vi "Read DC Output.vi"(8 "error in (no error)":errorcluster, 11 "VISA resource name":refnum<visa-resource-name>) -> (0 "error out":errorcluster, 1 "Actual DC Current Level (A)":dbl format="%.4g", 2 "Actual DC Voltage Level (V)":dbl format="%.4g", 3 "VISA resource name out":refnum<visa-resource-name>)   [LabVIEW 2015, in "BK Precision 983X Series.lvlib"]
doc: "Returns the actual DC voltage level and actual DC current level."
uses:
  <instrlib>/BK Precision 983X Series/BK Precision 983X Series.lvlib
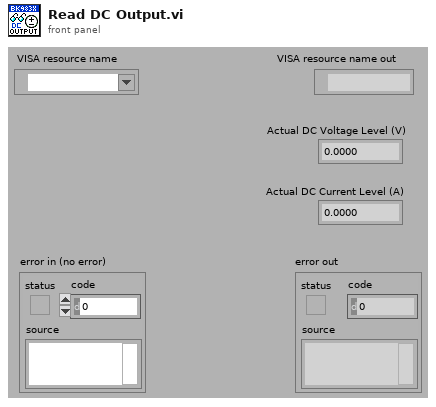
[diagram p1: front panel]
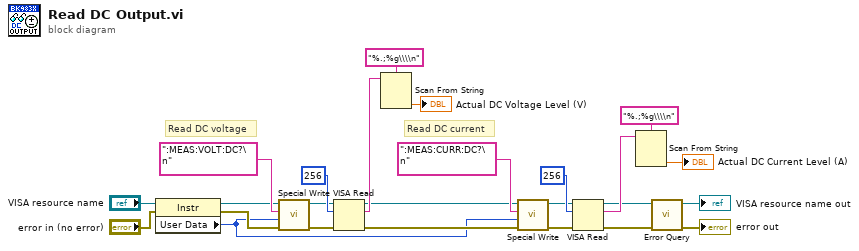
[diagram p0: block diagram]
diagram:
  # "Read DC current"
  # "Read DC voltage"
  n1 = property class="Instr"(reference="VISA resource name", error in="error in (no error)") -> (reference out=w14:refnum<visa-resource-name>, error out=w13:errorcluster, "User Data"=w5:u32)
  n2 = call <instrlib>:"Special Write.vi"("error in (no error)"=w13, "Delay (0 ms)"=w5, "Input String"=":MEAS:VOLT:DC?\n" ("format string"), "VISA resource name"=w14) -> ("error out"=w18:errorcluster, "VISA resource name out"=w19:refnum<visa-resource-name>)  [unwired: 6 in]
  n3 = VISA Read(VISA resource name=w19, byte count=u32 256, error in (no error)=w18) -> (VISA resource name out=w7:refnum<visa-resource-name>, read buffer=w22:string, error out=w6:errorcluster)  [unwired: 1 out]
  n4 = Scan From String(format string="%.;%g\\\\n", input string=w22) -> (output 1=→"Actual DC Voltage Level (V)":dbl)  [unwired: 3 in, 3 out]
  n5 = call <instrlib>:"Special Write.vi"("error in (no error)"=w6, "Delay (0 ms)"=w5, "Input String"=":MEAS:CURR:DC?\n" ("format string"), "VISA resource name"=w7) -> ("error out"=w9:errorcluster, "VISA resource name out"=w10:refnum<visa-resource-name>)  [unwired: 6 in]
  n6 = VISA Read(VISA resource name=w10, byte count=u32 256, error in (no error)=w9) -> (VISA resource name out=w3:refnum<visa-resource-name>, read buffer=w11:string, error out=w4:errorcluster)  [unwired: 1 out]
  n7 = Scan From String(format string="%.;%g\\\\n", input string=w11) -> (output 1=→"Actual DC Current Level (A)":dbl)  [unwired: 3 in, 3 out]
  n8 = call <instrlib>:"Error Query.vi"("error in (no error)"=w4, "VISA resource name"=w3) -> ("error out"=→"error out":errorcluster, "VISA resource name out"=→"VISA resource name out":refnum<visa-resource-name>)  [unwired: 6 in, 2 out]
